vi "Get Font .NET.vi"(11 "Font in":refnum<class "Font.lvclass">) -> (2 "Font .NET":refnum<k24>, 3 "Font out":refnum<class "Font.lvclass">)   [LabVIEW 2024, in "Font.lvclass"]
uses:
  Font.lvclass
  Font.lvclass/Font.ctl
  System.Drawing
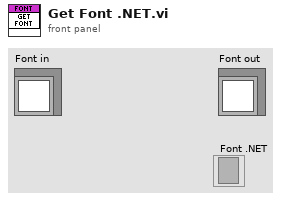
[diagram p1: front panel]
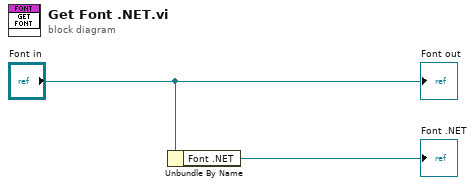
[diagram p0: block diagram]
diagram:
  n1 = Unbundle By Name("Font in") -> ("Font .NET"=→"Font .NET":refnum<k24>)
  "Font out" <- "Font in"
